vi "setUp.vi"(8 "error in (no error)":errorcluster, 11 "Test Runner.Collection in":refnum<class "Test Runner.Collection.lvclass">) -> (0 "error out":errorcluster, 3 "Test Runner.Collection out":refnum<class "Test Runner.Collection.lvclass">)   [LabVIEW 2013, in "Caraya.lvlib" / "Test Runner.Collection.lvclass"]
uses:
  Test Runner.Collection.lvclass
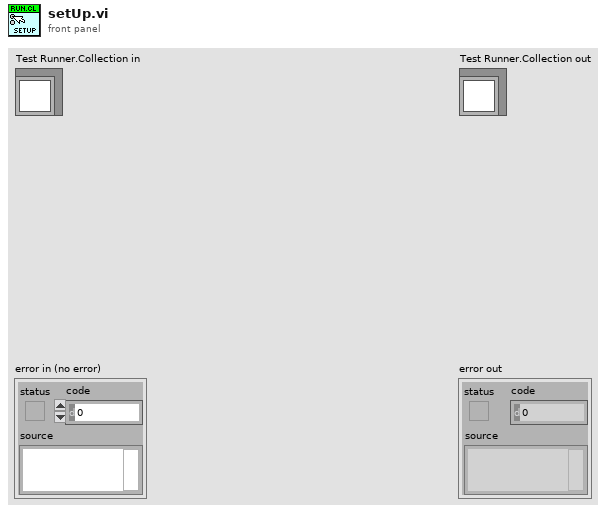
[diagram p1: front panel]
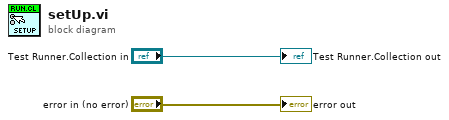
[diagram p0: block diagram]
diagram:
  "error out" <- "error in (no error)"
  "Test Runner.Collection out" <- "Test Runner.Collection in"
